vi "TDMS Viewer.vi"() -> ()   [LabVIEW 2015, in "Exposure Process.lvlib"]
uses:
  Exposure Process.lvlib
panel:
  in  "file path":path=path "C:/123/TLCD62/TDMS/TLCD62_20171121111508.tdms"
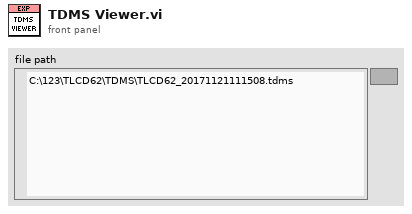
[diagram p1: front panel]
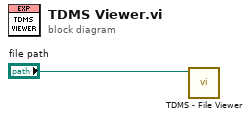
[diagram p0: block diagram]
diagram:
  n1 = call <vilib>:"TDMS - File Viewer.vi"("file path"="file path") -> ()  [unwired: 5 in, 2 out]
